vi "Q8381 Sole Header Off.vi"(0 "Row Data":string, 1 "Header\nPosition":u16, 2 "Header Length":u16=4) -> (3 "Header":string, 4 "Data Length":u32, 5 "Head-Off Data Length":u16, 6 "Head-Off Data":string)   [LabVIEW 2017]
doc: "Remove header from data string with sole header. Rest of data are out."
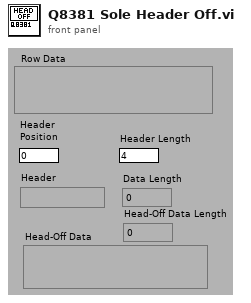
[diagram p1: front panel]
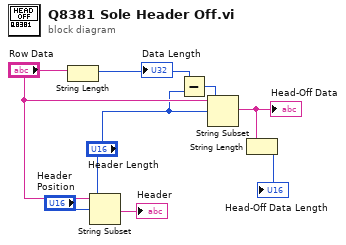
[diagram p0: block diagram]
diagram:
  n1 = String Length(string="Row Data") -> (length=w8:i32)
  "Data Length" <- w8
  n2 = String Subset(string="Row Data", offset (0)="Header\nPosition", length (rest)="Header Length") -> (substring=→"Header":string)
  n3 = Subtract(x=w8, y="Header Length") -> (x-y=w3:i32)
  n4 = String Subset(string="Row Data", offset (0)="Header Length", length (rest)=w3) -> (substring=w2:string)
  "Head-Off Data" <- w2
  n5 = String Length(string=w2) -> (length=→"Head-Off Data Length":i32)
